vi "example_01_get_commit_hash.vi"() -> ()   [LabVIEW 2015, in "lv-bin-git.lvlib" / "v1.lvlib"]
uses:
  v1.lvlib
  <userlib>/antonio-alexander/lv-bin/lv-bin/public/api/v1/advanced/add_data_path_multiple.vi
  <userlib>/antonio-alexander/lv-bin/lv-bin/public/api/v1/v1.lvlib
panel:
  out "commit_hash":string
  out "error out":errorcluster
  in  "bin_path":path
  in  "source_folder":path
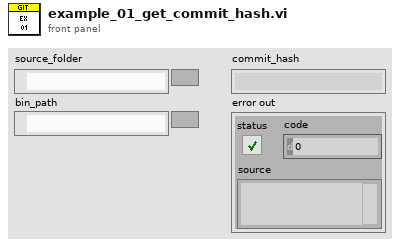
[diagram p1: front panel]
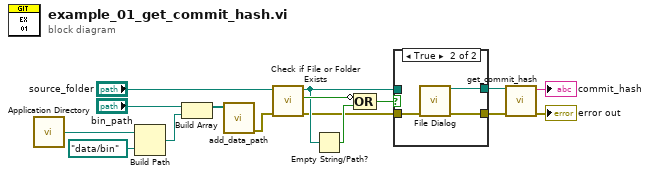
[diagram p0: block diagram]
diagram:
  n1 = call <vilib>:"Application Directory.vi"() -> ("Application Directory"=w12:path)
  n2 = Build Path(base path=w12, name or relative path=path "data/bin" ("Application Directory")) -> (appended path=w13:path)
  n3 = Build Array("bin_path", w13) -> (w14:path[])
  n4 = call-poly <userlib>:"add_data_path.vi"("path_to_add []"=w14) -> ("error out"=w8:errorcluster)  [unwired: 10 in]
  n5 = call <vilib>:"Check if File or Folder Exists.vi"("error in (no error)"=w8, "path"="source_folder") -> ("error out"=w6:errorcluster, "file or folder exists?"=w10:bool, "dup path"=w7:path)  [unwired: 7 in]
  n6 = Empty String/Path?(string/path=w7) -> (empty?=w9:bool)
  n7 = Compound Arithmetic op=OR(invert w10, w9) -> (w5:bool)
  n8 = case shown="True" w5 {
    tunnel: w7 -> [w18 _]
    tunnel: w6 -> [w17 w21]
    tunnel: [w17 w20] -> w4
    tunnel: [w18 w19] -> w3
    frame False {
    }
    frame True {
      n9 = call "File Dialog"("error in"=w21) -> ("selected path"=w19:path, "error out"=w20:errorcluster)  [unwired: 11 in, 2 out]
    }
  }
  n10 = call "get_commit_hash.vi"("error in (no error)"=w4, "path"=w3) -> ("error out"=→"error out":errorcluster, "commit_hash"=→"commit_hash":string)  [unwired: 8 in]
